vi "New Layout-polymorphic.vi"   [LabVIEW 2021, in "Appearance Actor.lvlib" / "Layout.lvclass"]
uses:
  Layout.lvclass
  Predifined Layout/Top Window/Top Window.lvclass
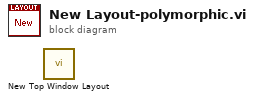
[diagram p0: block diagram]
diagram:
  n1 = call "New Top Window Layout.vi"() -> ()  [unwired: 10 in, 2 out]
